vi "Set Operational Mode.vi"(7 "Box ID":u8, 8 "error in (no error)":errorcluster, 9 "Precision Mode":bool, 10 "PID Disable":bool, 11 "Ethernet in":refnum<class "ENET_BS1201.lvclass">) -> (0 "error out":errorcluster, 3 "Ethernet out":refnum<class "ENET_BS1201.lvclass">)   [LabVIEW 2021, in "BS120x Driver.lvlib" / "ENET_BS1201.lvclass"]
uses:
  ENET_BS1201.lvclass
  C:/Users/Public/Documents/Projects/7100-00109 SW BS1201 LV Driver/trunk/source/ENET_BS120x/ENET_BS120x.lvclass
  ENET_BS1201.lvclass/ENET_BS1201.ctl
  ENET_BS120x/ENET_BS120x.lvclass
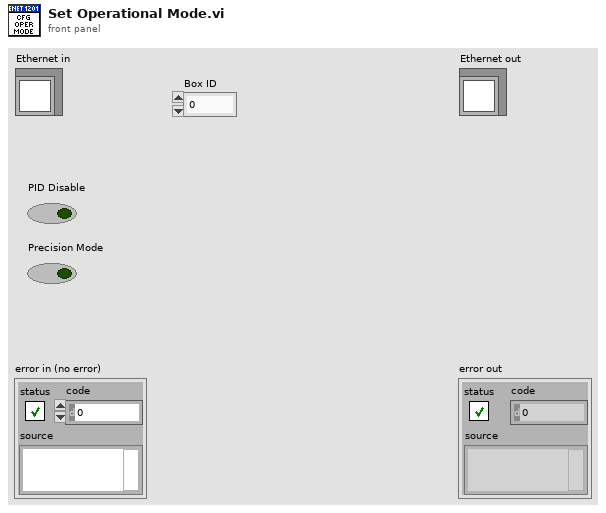
[diagram p1: front panel]
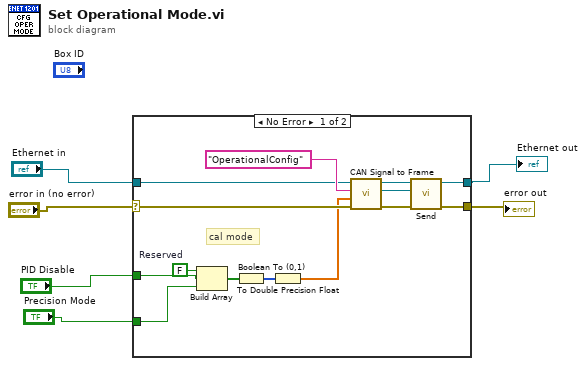
[diagram p0: block diagram]
diagram:
  n1 = case shown="No Error" "error in (no error)" {
    selector: "error in (no error)" -> [w15 w21]
    tunnel: [w16 w21] -> w1
    tunnel: "Ethernet in" -> [w14 w22]
    tunnel: [w13 w22] -> w2
    tunnel: "PID Disable" -> [w9 _]
    tunnel: "Precision Mode" -> [w8 _]
    frame No Error {
      w7 = FALSE  # Reserved
      # "cal mode"
      n2 = Build Array(w7, w9, w8) -> (w11:bool[])
      n3 = Boolean To (0,1)(Boolean=w11) -> (0, 1=w12:i16[])
      n4 = To Double Precision Float(number=w12) -> (double precision float=w10:dbl[])
      n5 = call "CAN Signal to Frame.vi"("error in (no error)"=w15, "Data Array"=w10, "Frame"="OperationalConfig", "ENET in"=w14) -> ("error out"=w17:errorcluster, "Data"=w18:refnum<class "Data.lvclass">, "ENET out"=w19:refnum<class "ENET_BS1201.lvclass">)  [unwired: 5 in]
      n6 = call "Send.vi"("error in (no error)"=w17, "Data"=w18, "ENET in"=w19) -> ("error out"=w16:errorcluster, "ENET out"=w13:refnum<class "ENET_BS1201.lvclass">)  [unwired: 7 in]
    }
    frame Error {
    }
  }
  "error out" <- w1
  "Ethernet out" <- w2
